vi "Validate.vi"(8 "error in (no error)":errorcluster, 11 "Class in":refnum<class "AB_UI_Frmwk_Installer.lvclass">) -> (0 "error out":errorcluster, 3 "Class out":refnum<class "AB_UI_Frmwk_Installer.lvclass">)   [LabVIEW 2020, in "AB_UI_Frmwk_Installer.lvclass"]
uses:
  <vilib>/AppBuilder/IB_Classes/Installer/UI/AB_UI_Frmwk_Installer.lvclass
  <vilib>/AppBuilder/IB_Classes/Installer/Installer.lvclass
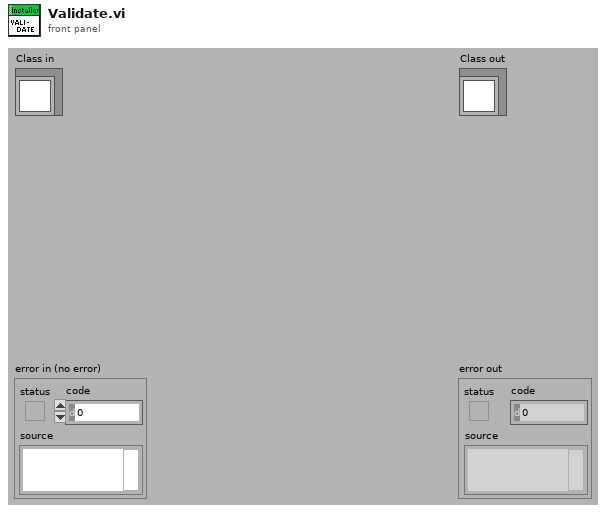
[diagram p1: front panel]
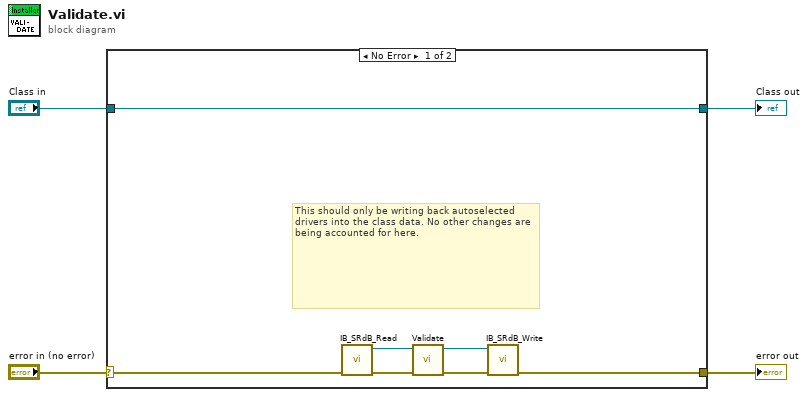
[diagram p0: block diagram]
diagram:
  n1 = case shown="No Error" "error in (no error)" {
    selector: "error in (no error)" -> [w10 w13]
    tunnel: [w5 w13] -> w1
    tunnel: [w11 w12] -> w4
    tunnel: "Class in" -> [w11 w12]
    frame No Error {
      # "This should only be writing back autoselected drivers into the class data. No other changes are being accounted for here."
      n2 = call <resource>:"IB_SRdB_Read.vi"("error in (no error)"=w10) -> ("error out"=w8:errorcluster, "installer out"=w9:refnum<class "Installer.lvclass">)  [unwired: 9 in]
      n3 = call-dynamic "Validate.vi"("error in (no error)"=w8, "Class in"=w9) -> ("error out"=w6:errorcluster, "Class out"=w7:refnum<class "Installer.lvclass">)  [unwired: 8 in]
      n4 = call <resource>:"IB_SRdB_Write.vi"("error in (no error)"=w6, "installer"=w7) -> ("error out"=w5:errorcluster)  [unwired: 9 out]
    }
    frame Error {
    }
  }
  "error out" <- w1
  "Class out" <- w4
